vi "Validade Column Names.vi"(8 "error in (no error)":errorcluster, 11 "ORM Scripter in":refnum<class "ORM Scripter.lvclass">) -> (0 "error out":errorcluster, 3 "ORM Scripter out":refnum<class "ORM Scripter.lvclass">)   [LabVIEW 2018, in "ORM Scripter.lvclass"]
uses:
  ORM Scripter.lvclass
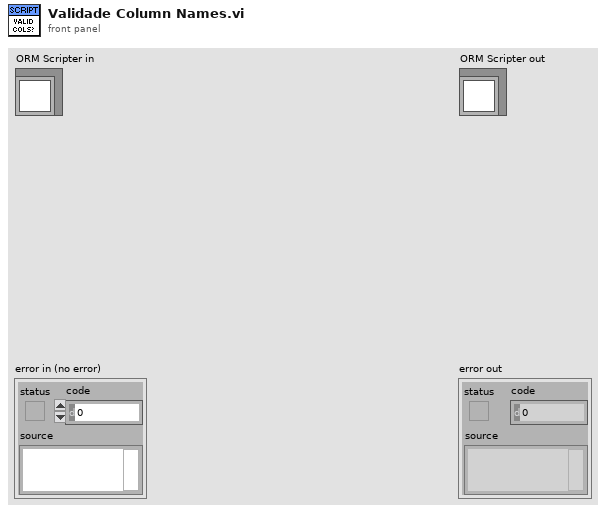
[diagram p1: front panel]
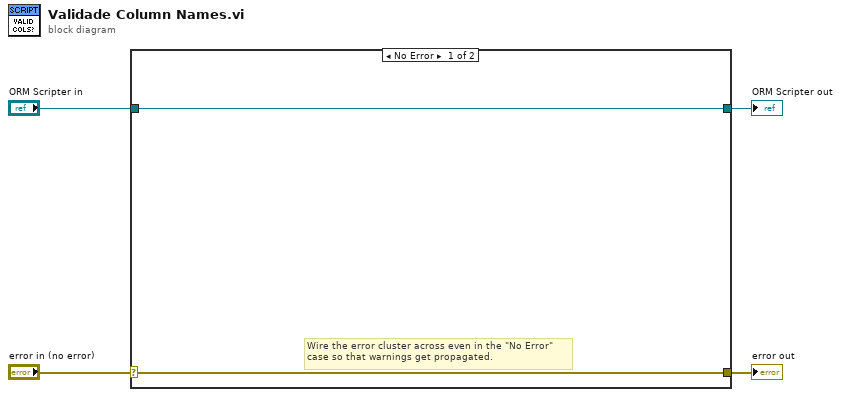
[diagram p0: block diagram]
diagram:
  n1 = case shown="No Error" "error in (no error)" {
    selector: "error in (no error)" -> [w5 w8]
    tunnel: [w5 w8] -> w3
    tunnel: [w6 w7] -> w1
    tunnel: "ORM Scripter in" -> [w6 w7]
    frame No Error {
      # "Wire the error cluster across even in the \"No Error\"\ncase so that warnings get propagated."
    }
    frame Error {
    }
  }
  "error out" <- w3
  "ORM Scripter out" <- w1
